vi "WD_Set_NULL_assemble_data.vi"(8 "error in (no error)":errorcluster, 11 "DBlink":string="Driver={ODBC Driver 17 for SQL Server};Server=localhost\\SQLEXPRESS;Database=ZDX201;UID=labview;PWD=Dsa@54137926") -> (0 "error out":errorcluster={"status"=TRUE, "code"=-2147217843, "source"="NI_Database_API.lvlib:DB Tools Open Connec (String).vi->WD_assemble_data.vi<ERR>ADO Error: 0x80040E4D\r\nException occured in Microsoft OLE DB Provider for ODBC Drivers: [Microsoft][ODBC Driver 17 for SQL Server][SQL Server]使用者 'labview' 的登入失敗。 in NI_Database_API.lvlib:DB Tools Open Connec (String).vi->WD_assemble_data.vi"}, 2 "Workplace: assemble":cluster{"條碼A":string, "條碼B":string}[](array[cluster]))   [LabVIEW 2019]
uses:
  <vilib>/addons/database/Connection.llb/DB Tools Open Connec (String).vi
  <vilib>/addons/database/Connection.llb/Conn Execute.vi
  <vilib>/addons/database/Recordset.llb/Rec Fetch Recordset Data (R).vi
  <vilib>/addons/database/Recordset.llb/Rec Destroy - Connection.vi
  <vilib>/addons/database/_DB Variant To Data/Database Variant To Data.xnode
  <vilib>/addons/database/NI_Database_API.lvlib
panel:
  out "查詢結果":string="SELECT [id]\n      ,[name]\n      ,[barcode A]\n      ,[barcode B]\n      ,[update_time]\n  FROM [ZDX201].[dbo].[workplace_data]\n  where id>0 and id<6\n  order by id"
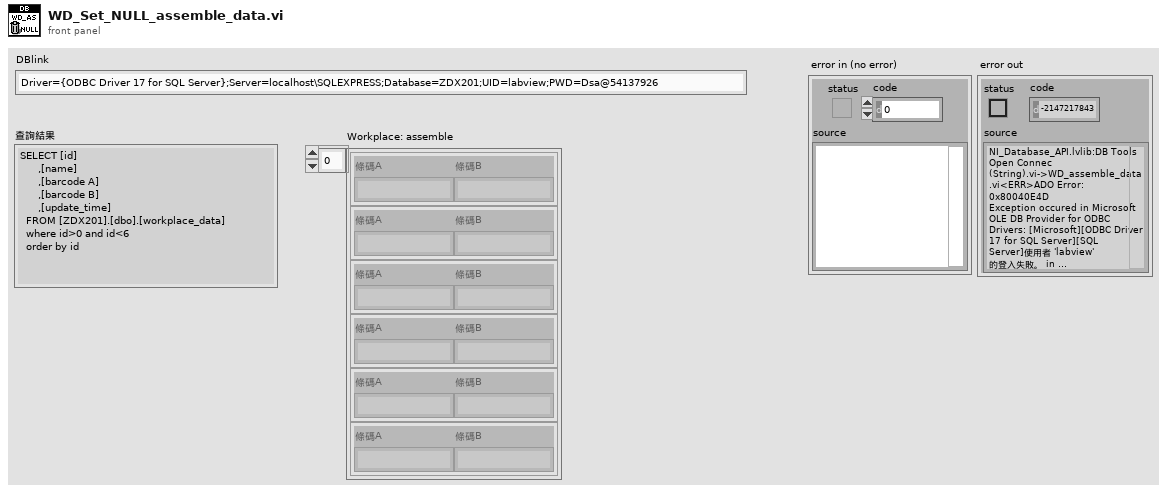
[diagram p1: front panel]
types:
  T1 = typedef "NI_Database_API.lvlib/Conn ObjectReference.ctl" = refnum<k1>
  T2 = typedef "NI_Database_API.lvlib/Rec ObjectReference.ctl" = refnum<k1>
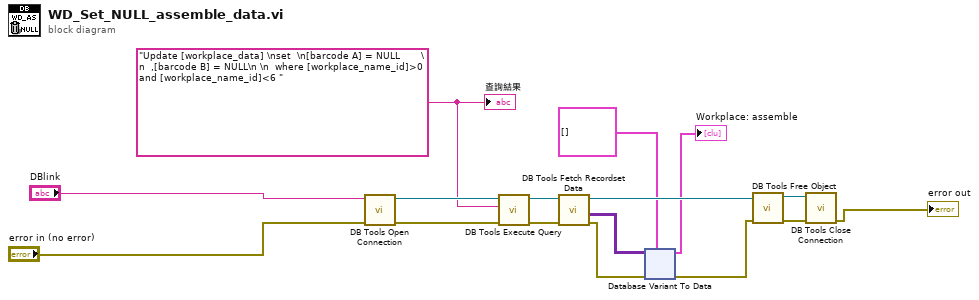
[diagram p0: block diagram]
diagram:
  w6 = "Update [workplace_data] \nset  \n[barcode A] = NULL       \n  ,[barcode B] = NULL\n \n  where [workplace_name_id]>0 and [workplace_name_id]<6 "
  n1 = call-poly <vilib>:"DB Tools Open Connection.vi"("error in (no error)"="error in (no error)", "connection information"="DBlink") -> ("error out"=w16:errorcluster, "connection reference"=w15:T1)  [unwired: 6 in]
  n2 = call-poly <vilib>:"DB Tools Execute Query.vi"("error in (no error)"=w16, "SQL query"=w6, "connection reference"=w15) -> ("error out"=w13:errorcluster, "recordset reference"=w14:T2)  [unwired: 5 in]
  n3 = call-poly <vilib>:"DB Tools Fetch Recordset Data.vi"("error in (no error)"=w13, "recordset reference"=w14) -> ("error out"=w8:errorcluster, "recordset data"=w7:variant[][], "recordset reference out"=w9:T2)  [unwired: 3 in]
  n4 = xnode "Database Variant To Data"("database variant"=w7, "error in (no error)"=w8, "type"=cluster{"條碼A":string, "條碼B":string}[] [] ("Workplace: assemble")) -> ("data"=→"Workplace: assemble":cluster{"條碼A":string, "條碼B":string}[], "error out"=w10:errorcluster)
  n5 = call-poly <vilib>:"DB Tools Free Object.vi"("error in (no error)"=w10, "recordset reference"=w9) -> ("error out"=w11:errorcluster, "connection reference"=w12:T1)  [unwired: 8 in]
  n6 = call <vilib>:"DB Tools Close Connection.vi"("error in (no error)"=w11, "connection reference"=w12) -> ("error out"=→"error out":errorcluster)  [unwired: 5 in]
  "查詢結果" <- w6
